vi "exercise 3-9.vi"() -> ()   [LabVIEW 2014]
panel:
  out "Warning Text":string
  out "Warning?":bool
  in  "Current Temp":dbl
  in  "Max Wind Speed":dbl
  in  "Current Wind Speed":dbl
  in  "Max Temp":dbl
  in  "Min Temp":dbl
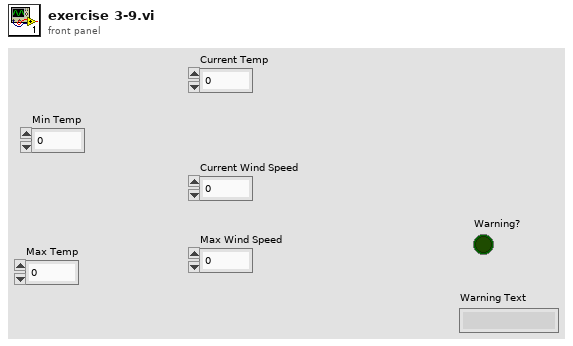
[diagram p1: front panel]
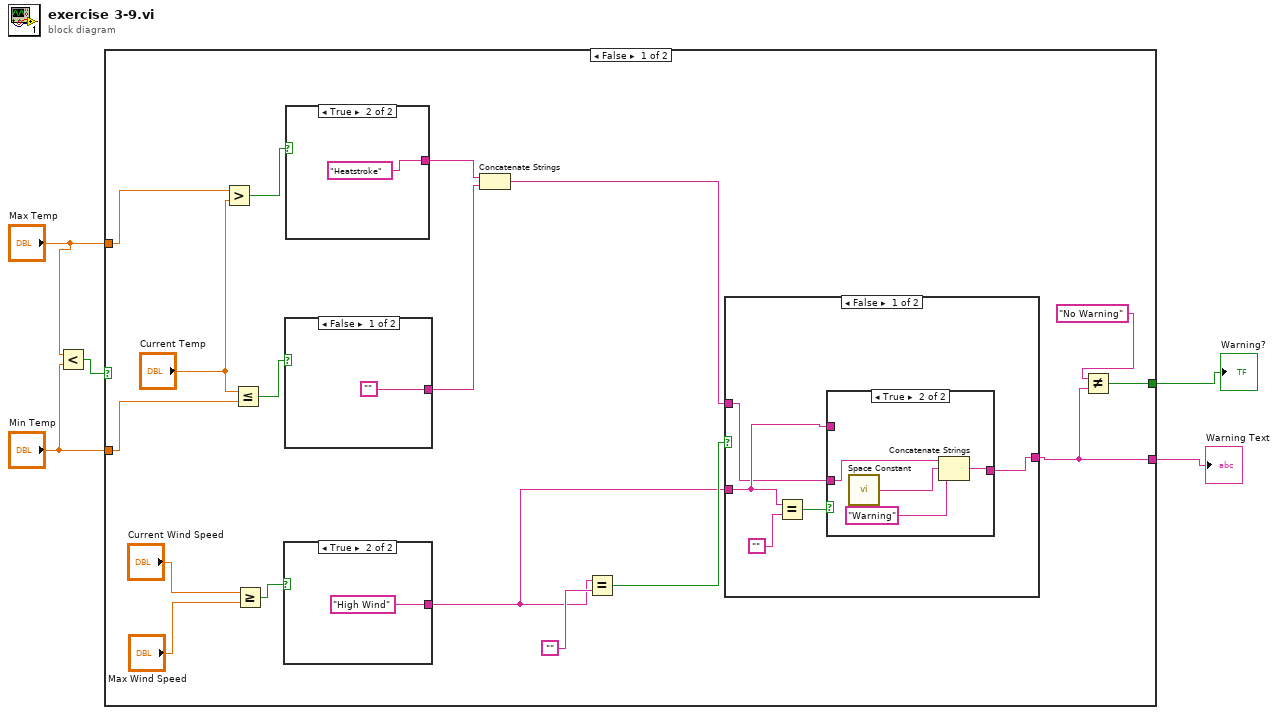
[diagram p0: block diagram]
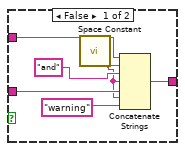
[diagram p2: hidden frame]
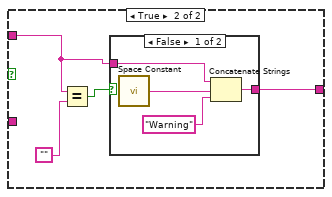
[diagram p3: hidden frame]
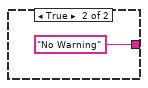
[diagram p4: hidden frame]
diagram:
  n1 = Less?(x="Max Temp", y="Min Temp") -> (x < y?=w3:bool)
  n2 = case shown="False" w3 {
    tunnel: "Max Temp" -> [w21 _]
    tunnel: "Min Temp" -> [w20 _]
    tunnel: [w6 _] -> w1
    tunnel: [w7 _] -> w2
    frame False {
      n3 = Greater?(x=w21, y="Current Temp") -> (0:w19:bool)
      n4 = Less Or Equal?(x="Current Temp", y=w20) -> (x <= y?=w18:bool)
      n5 = Greater Or Equal?(x="Current Wind Speed", y="Max Wind Speed") -> (x >= y?=w17:bool)
      n6 = case shown="True" w17 {
        tunnel: [_ "High Wind"] -> w9
        frame False {
        }
        frame True {
        }
      }
      n7 = case shown="False" w18 {
        tunnel: ["" _] -> w13
        frame False {
        }
        frame True {
        }
      }
      n8 = case shown="True" w19 {
        tunnel: [_ "Heatstroke"] -> w14
        frame False {
        }
        frame True {
        }
      }
      n9 = Concatenate Strings(w14, w13) -> (w12:string)
      n10 = Equal?(x=w9, y="") -> (x = y?=w11:bool)
      n11 = case shown="False" w11 {
        tunnel: w12 -> [w24 w39]
        tunnel: w9 -> [w25 _]
        tunnel: [w23 w38] -> w6
        frame False {
          n12 = Equal?(x=w25, y="") -> (x = y?=w27:bool)
          n13 = case shown="True" w27 {
            tunnel: w25 -> [w33 _]
            tunnel: w24 -> [w32 w37]
            tunnel: [w28 w34] -> w23
            frame False {
              n14 = call <vilib>:"Space Constant.vi"() -> ("String"=w30:string)
              n15 = Concatenate Strings(w33, w30, "and", w30, w32, w30, "warning") -> (w28:string)
            }
            frame True {
              n16 = call <vilib>:"Space Constant.vi"() -> ("String"=w36:string)
              n17 = Concatenate Strings(w37, w36, "Warning") -> (w34:string)
            }
          }
        }
        frame True {
          n18 = Equal?(x=w39, y="") -> (x = y?=w40:bool)
          n19 = case shown="False" w40 {
            tunnel: w39 -> [w43 _]
            tunnel: [w42 "No Warning"] -> w38
            frame False {
              n20 = call <vilib>:"Space Constant.vi"() -> ("String"=w44:string)
              n21 = Concatenate Strings(w43, w44, "Warning") -> (w42:string)
            }
            frame True {
            }
          }
        }
      }
      n22 = Not Equal?(x="No Warning", y=w6) -> (x != y?=w7:bool)
    }
    frame True {
    }
  }
  "Warning?" <- w2
  "Warning Text" <- w1
